vi "Find Non Zero Points.vi"(8 "error in (no error)":errorcluster, 11 "Greyscale Image-Source in":T2) -> (0 "error out":errorcluster, 3 "Non Zero Points":T1[](array[typedef]))   [LabVIEW 2020, in "image.lvlib"]
doc: "Get the points in the image which are non-zero."
uses:
  image.lvlib
  Greyscale Image.ctl
  common/Image Point (Integer).ctl
  common/common.lvlib
  common/bin/gartoolkit_32-1.dll
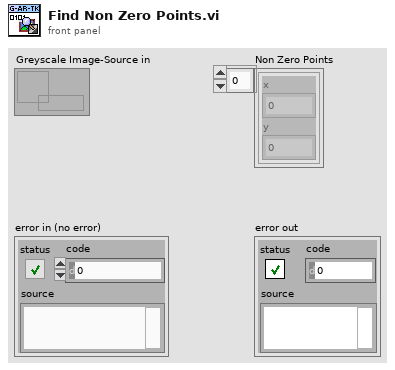
[diagram p1: front panel]
types:
  T1 = typedef "common.lvlib/Image Point (Integer).ctl" = cluster{"x":i32, "y":i32}
  T2 = typedef "image.lvlib/Greyscale Image.ctl" = refnum<data-value>
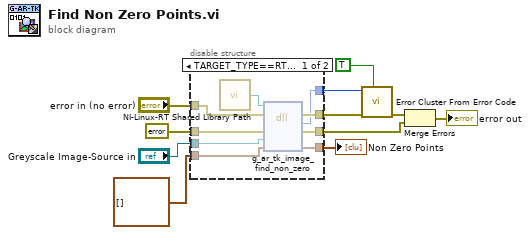
[diagram p0: block diagram]
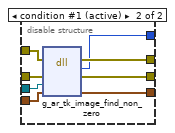
[diagram p2: hidden frame]
diagram:
  n1 = disable-structure shown="TARGET_TYPE==RT&&OS==Linux" {
    disable-tunnel: "error in (no error)" -> [w20 w28]
    disable-tunnel: errorcluster {"status"=FALSE, "code"=0, "source"=""} ("error constant") -> [w19 w27]
    disable-tunnel: "Greyscale Image-Source in" -> [w18 w26]
    disable-tunnel: T1[] [] ("Array") -> [w17 w25]
    disable-tunnel: [w16 w24] -> w5
    disable-tunnel: [w15 w23] -> w4
    disable-tunnel: [w14 w22] -> w3
    disable-tunnel: [w13 w21] -> w2
    frame condition #0 {
      n2 = call "NI-Linux-RT Shared Library Path.vi"() -> ("Path"=w12:path)
      n3 = dll-call lib="?" fn="g_ar_tk_image_find_non_zero" ("g_ar_toolkit.*.*:g_ar_tk_image_in_range")(path in=w12, error in=w20, "error_cluster"=w19, "EDVR src"=w18, "points"=w17) -> (error out=w16:errorcluster, "MgErr"=w15:i32, "error_cluster"=w14:errorcluster, "points"=w13:T1[])  [unwired: 2 in, 1 out]
    }
    frame condition #1 (active) {
      n4 = dll-call lib="C:/serenial/lib/g-augmented-reality-toolkit/LabVIEW/common/bin/gartoolkit_*-1.*" fn="g_ar_tk_image_find_non_zero" ("g_ar_toolkit.*.*:g_ar_tk_image_in_range")(error in=w28, "error_cluster"=w27, "EDVR src"=w26, "points"=w25) -> (error out=w24:errorcluster, "MgErr"=w23:i32, "error_cluster"=w22:errorcluster, "points"=w21:T1[])  [unwired: 3 in, 1 out]
    }
  }
  "Non Zero Points" <- w2
  n5 = call <vilib>:"Error Cluster From Error Code.vi"("show call chain? (False)"=TRUE, "error in (no error)"=w5, "error code (0)"=w4) -> ("error out"=w10:errorcluster)  [unwired: 6 in]
  n6 = Merge Errors(w10, w3) -> (→"error out":errorcluster)
